vi "ForceBalanceServer.vi"() -> ()   [LabVIEW 2017]
uses:
  <vilib>/Platform/TimedLoop/XDataNode/timing_clust.ctl
  <vilib>/Platform/TimedLoop/XDataNode/nitl_modes.ctl
  <vilib>/Platform/TimedLoop/XDataNode/wakeup.ctl
  <vilib>/Analysis/baseanly.llb/A x Vector.vi
  <vilib>/platform/TimedLoop/XDataNode/XDataNode.xnode
  <vilib>/Platform/TimedLoop/XDataNode/XDNodeRunTimeDep.lvlib
  <vilib>/Analysis/NI_AALBase.lvlib
panel:
  out "Mz":dbl
  out "My":dbl
  out "Mx":dbl
  out "Fz":dbl
  out "Fy":dbl
  out "Fx":dbl
  in  "Stop Button":bool
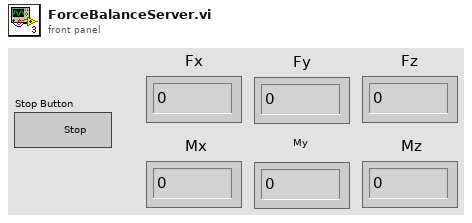
[diagram p1: front panel]
types:
  T1 = typedef "XDNodeRunTimeDep.lvlib/timing_clust.ctl" = cluster{"Expected End [f-1]":u64, "Actual End [f-1]":u64, "Finished Late? [f-1]":bool, "Expected End [i-1]":u64, "Actual End [i-1]":u64, "Finished Late? [i-1]":bool, "Expected Start [i]":u64, "Actual Start [i]":u64, "Expected Start [f]":u64, "Actual Start [f]":u64, "Source Name":string, "Structure Name":string, "Period":i64, "Deadline":i64, "Offset":i64, "Start":i64, "Priority":i32, "Timeout":i32, "Mode":T2, "Wakeup Reason":T3, "Error":errorcluster, "Source Type":string, "Secondary Source Type":string, "Global End Time":u64, "Global Start Time":u64, "Frame Duration":u64, "Iteration Duration":u64, "Assigned CPU":i32, "I/O Scan Engine Mode":u32}
  T2 = typedef "XDNodeRunTimeDep.lvlib/nitl_modes.ctl" = enum32{"No Change", "Process missed periods, maintain original phase", "Discard missed periods, maintain original phase", "Process missed periods, ignore original phase", "Discard missed periods, ignore original phase"}
  T3 = typedef "XDNodeRunTimeDep.lvlib/wakeup.ctl" = enum32{"Normal", "Aborted", "Asynchronous wakeup", "Timing source error", "Timed loop error", "Timeout"}
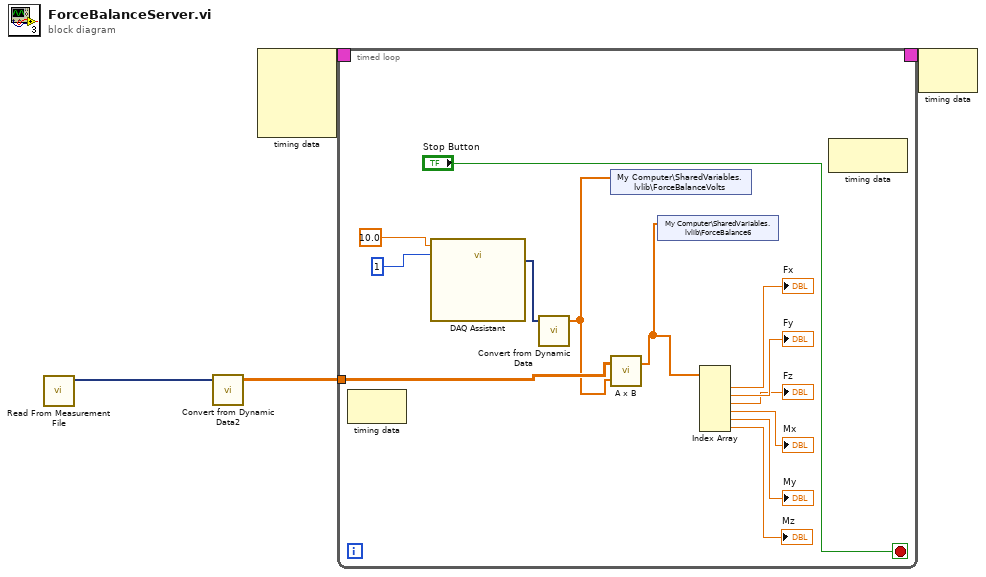
[diagram p0: block diagram]
diagram:
  n1 = call "Read From Measurement File"() -> ("Signals"=w2:dynamicdata)  [unwired: 6 in, 5 out]
  n2 = call "Convert from Dynamic Data2"("Dynamic Data Type"=w2) -> ("Array"=w1:dbl[][])  [unwired: 3 in]
  n3 = node-c288() -> (w4:T1)  [unwired: 4 in]
  n4 = timed-loop {
    timing: w4 -> [_]
    timing-out: [_] -> w3
    tunnel: w1 -> [w7]
    stop <- "Stop Button" stop-if-true
    n5 = node-c288() -> ()  [unwired: 1 in, 1 out]
    n6 = call "DAQ Assistant"("rate"=10.0, "number of samples"=1) -> ("data"=w14:dynamicdata)  [unwired: 14 in, 3 out]
    n7 = call "Convert from Dynamic Data"("Dynamic Data Type"=w14) -> ("Array"=w5:dbl[])  [unwired: 3 in]
    n8 = shared-variable "My Computer\\SharedVariables.lvlib\\ForceBalanceVolts"(w5) -> ()  [unwired: 1 in, 1 out]
    n9 = call-poly <vilib>:"A x B.vi"("Vector"=w5, "A"=w7) -> ("A x Vector"=w6:dbl[])  [unwired: 1 out]
    n10 = shared-variable "My Computer\\SharedVariables.lvlib\\ForceBalance6"(w6) -> ()  [unwired: 1 in, 1 out]
    n11 = Index Array(array=w6) -> (element #1=→"Fx":dbl, element #2=→"Fy":dbl, element #3=→"Fz":dbl, element #4=→"Mx":dbl, element #5=→"My":dbl, element #6=→"Mz":dbl)  [unwired: 6 in]
    n12 = node-c288() -> ()  [unwired: 1 in, 1 out]
  }
  n13 = node-c288(w3) -> ()  [unwired: 1 out]
